vi "Write Element of PHI.vi"(8 "error in (no error)":errorcluster, 9 "Real Matrix Element":dbl, 10 "indices":i32[](array[numeric]), 11 "Kalman Filter in":refnum<class "Kalman Filter.lvclass">) -> (0 "error out":errorcluster, 3 "Kalman Filter out":refnum<class "Kalman Filter.lvclass">)   [LabVIEW 2014, in "Observer Library.lvlib" / "Kalman Filter.lvclass"]
uses:
  Kalman Filter.lvclass
  Kalman Filter.lvclass/Kalman Filter.ctl
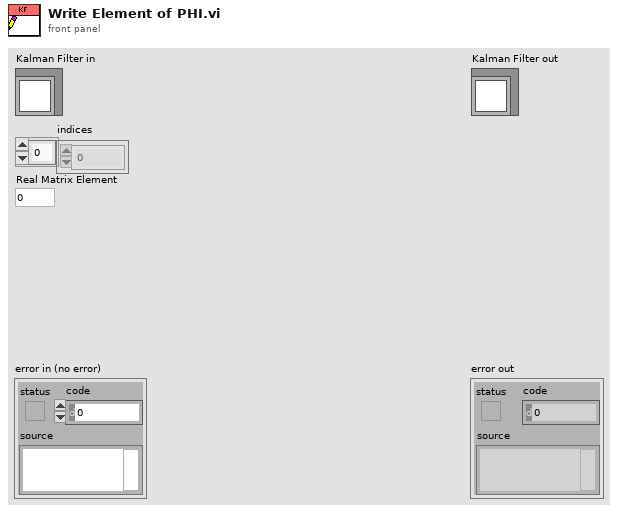
[diagram p1: front panel]
types:
  T1 = typedef "NI_Matrix.lvlib/RealMatrix.ctl" = dbl[][]
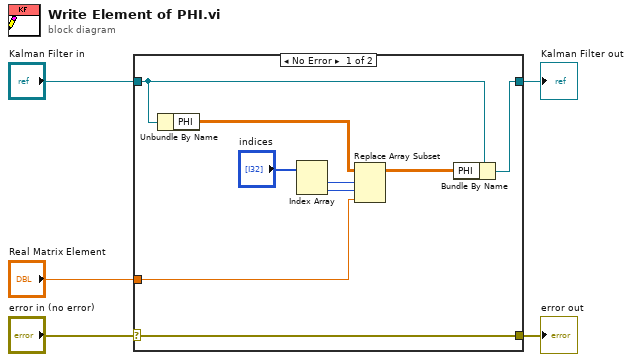
[diagram p0: block diagram]
diagram:
  n1 = case shown="No Error" "error in (no error)" {
    selector: "error in (no error)" -> [w14 w15]
    tunnel: [w14 w15] -> w4
    tunnel: [w13 w16] -> w2
    tunnel: "Kalman Filter in" -> [w6 w16]
    tunnel: "Real Matrix Element" -> [w7 _]
    frame No Error {
      n2 = Unbundle By Name(w6) -> ("PHI"=w8:T1)
      n3 = Index Array(array="indices") -> (element #1=w10:i32, element #2=w9:i32)  [unwired: 2 in]
      n4 = Replace Array Subset(array=w8, new element=w7, index (row)=w10, index (col)=w9) -> (w12:T1)
      n5 = Bundle By Name(cluster=w6, "PHI"=w12) -> (w13:refnum<class "Kalman Filter.lvclass">)
    }
    frame Error {
    }
  }
  "error out" <- w4
  "Kalman Filter out" <- w2
